vi "Get Message Transport Event Registration.vi"(8 "error in (no error)":errorcluster, 11 "Message Transport Event in":refnum<class "Message Transport Event.lvclass">) -> (0 "error out":errorcluster, 1 "Event":refnum<user-event>, 2 "Event Registration Refnum":refnum<event-registration>, 3 "Message Transport Event out":refnum<class "Message Transport Event.lvclass">)   [LabVIEW 2016, in "Stream Mediator.lvlib" / "Message Transport Event.lvclass"]
doc: "--\nCopyright © 2017 Composed SystemsI All rights reserved.\n\nAuthor: Jon McBee <jon.mcbee@composed.io>\n\nThis library is provided \"AS IS\" ,WITHOUT WARRANTIES OR\nCONDITIONS OF ANY KIND, either express or implied.\n\nComposed Systems -- composed.io\n\nStream 0.0.1.1\nJon McBee - Composed Systems\nCopyright (c) 2017, Composed Systems"
uses:
  <userlib>/Composed Systems/Stream/Mediator/Classes/Message Transport Event/Message Transport Event.lvclass
  <userlib>/Composed Systems/Stream/Mediator/Classes/Message Interface/Message Interface.lvclass
  <userlib>/Composed Systems/Stream/Mediator/Classes/Message Transport Event/Message Transport Event.lvclass/Message Transport Event.ctl
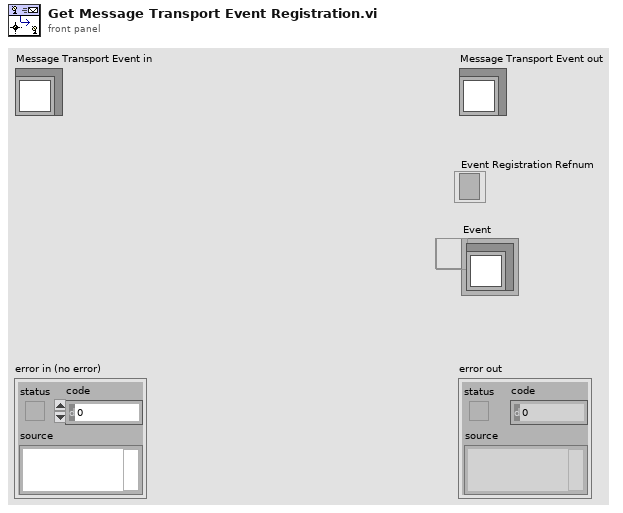
[diagram p1: front panel]
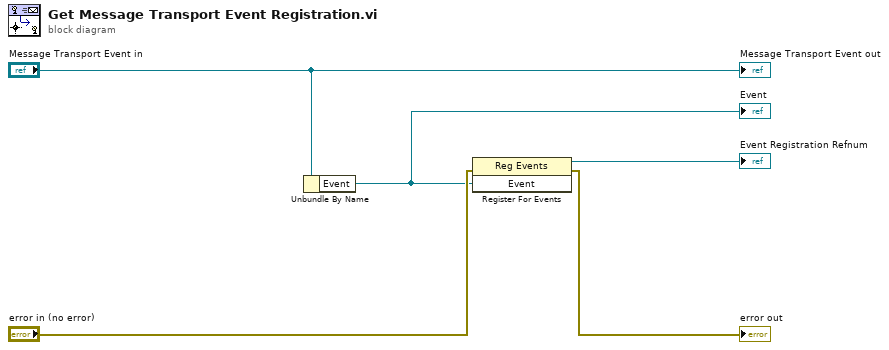
[diagram p0: block diagram]
diagram:
  n1 = Unbundle By Name("Message Transport Event in") -> ("Event"=w1:refnum<user-event>)
  "Event" <- w1
  n2 = register-events(error in="error in (no error)", w1) -> (reference out=→"Event Registration Refnum":refnum<event-registration>, error out=→"error out":errorcluster)  [unwired: 1 in]
  "Message Transport Event out" <- "Message Transport Event in"
